vi "main.vi-simplified.vi"() -> ()   [LabVIEW 2023]
uses:
  state-machine-states.ctl
  sub-vi/csv-file-logging/filepath-selection.ctl
  tab-control-states.ctl
  <vilib>/DAQmx/read.llb/DAQmx Read (Analog DBL 1Chan 1Samp).vi
  <vilib>/DAQmx/create/channels.llb/DAQmx Create Channel (AI-Temperature-Thermocouple).vi
  <vilib>/DAQmx/miscellaneous.llb/DAQmx Fill In Error Info.vi
  bronkhorst_flow-bus/Bronkhorst FLOW-BUS/Public/Data/Measure/Read Measure (Direct).vi
  bronkhorst_flow-bus/Bronkhorst FLOW-BUS/Bronkhorst FLOW-BUS.lvlib
panel:
  in  "Datalogging options":T1={"Include Timestamp"=TRUE, "Include milliseconds"=FALSE, "data-precision"=3}
  in  "Stop":bool
  in  "pause":bool
  in  "exit":bool
  out "state":T2
  out "error out":errorcluster
  out "Status":string
  in  "Tab Control":enum32{"setup", "run", "graphs", "errors"}(tab)
  in  "Simulate Hardware":bool
  in  "Start":bool
  in  "MFC 1":refnum<visa-resource-name>="COM31"
  in  "MFC 2":refnum<visa-resource-name>="COM32"
  in  "MFM 3":refnum<visa-resource-name>="COM5"
  in  "MFM 4":refnum<visa-resource-name>="COM6"
  in  "TC1 Channel":tag="cDAQ1Mod1/ai0"
  in  "TC2 Channel":tag="cDAQ1Mod1/ai1"
  in  "Filepath Selection":T3={"Log Filepath Source"=enum."Application Relative (Auto)", "Log File Path (Manual)"=path "C:/Users/dheard/Documents/0002-labview-projects/ammonia-absorbsion-rig/data", "Log File Folder Name"="data", "log file name"="log", "Include Date in Filename"=TRUE, "Include Time in Filename"=TRUE}
  out "appended path for log file":path
  out "MFM4 (ml/min) 2":dbl caption="Measure Percentage"
  out "MFM3 (ml/min)":dbl caption="Measure Percentage"
  out "TC1 (degC)":dbl format="%0.2f"
  out "TC2 (degC)":dbl format="%0.2f"
  out "MFM Sensor History":dbl[][](graph)
  out "Temperature Sensor History":dbl[][](graph)
  out "errors":errorcluster
  in  "Clear Errors":bool
  # "Usage Instructions:\n\n1. Select \"setup\" tab, ensure correct \n    COM port & Channel for each device\n\n2. To start Data Aquisition press \"Start\" button\n\n3. View Graphs in \"graphs\" tab\n\n4. Pause and Unpause data aquisition with \"pause\" button\n\n5. To export data to Excel, right click on topmost graph view \n     and select:\n     - \"Export\" -> \"Export  Data to Excel\"\n     - Name & Save Excel file\n        (Note: All data will be exported not just \"active\" plots)\n\n\n6. To Clear sensor history press \"Stop\" button\n     - While stopped, setup controls are available\n\n7. To Exit program, click \"Exit\" Button\n\n8. If Error shows, attempt to remedy error then press\n     \"clear error\" button. Program will revert to Setup"
  # "Column Temp"
  # "Heater Temp"
  # "Percentage"
  # "Gas  \nOut"
  # "Nitrogen \nIn"
  # "Ammonia \nIn"
  # "Gas  \nOut"
  # "MFC2"
  # "MFM4"
  # "MFM3"
  # "MFC1"
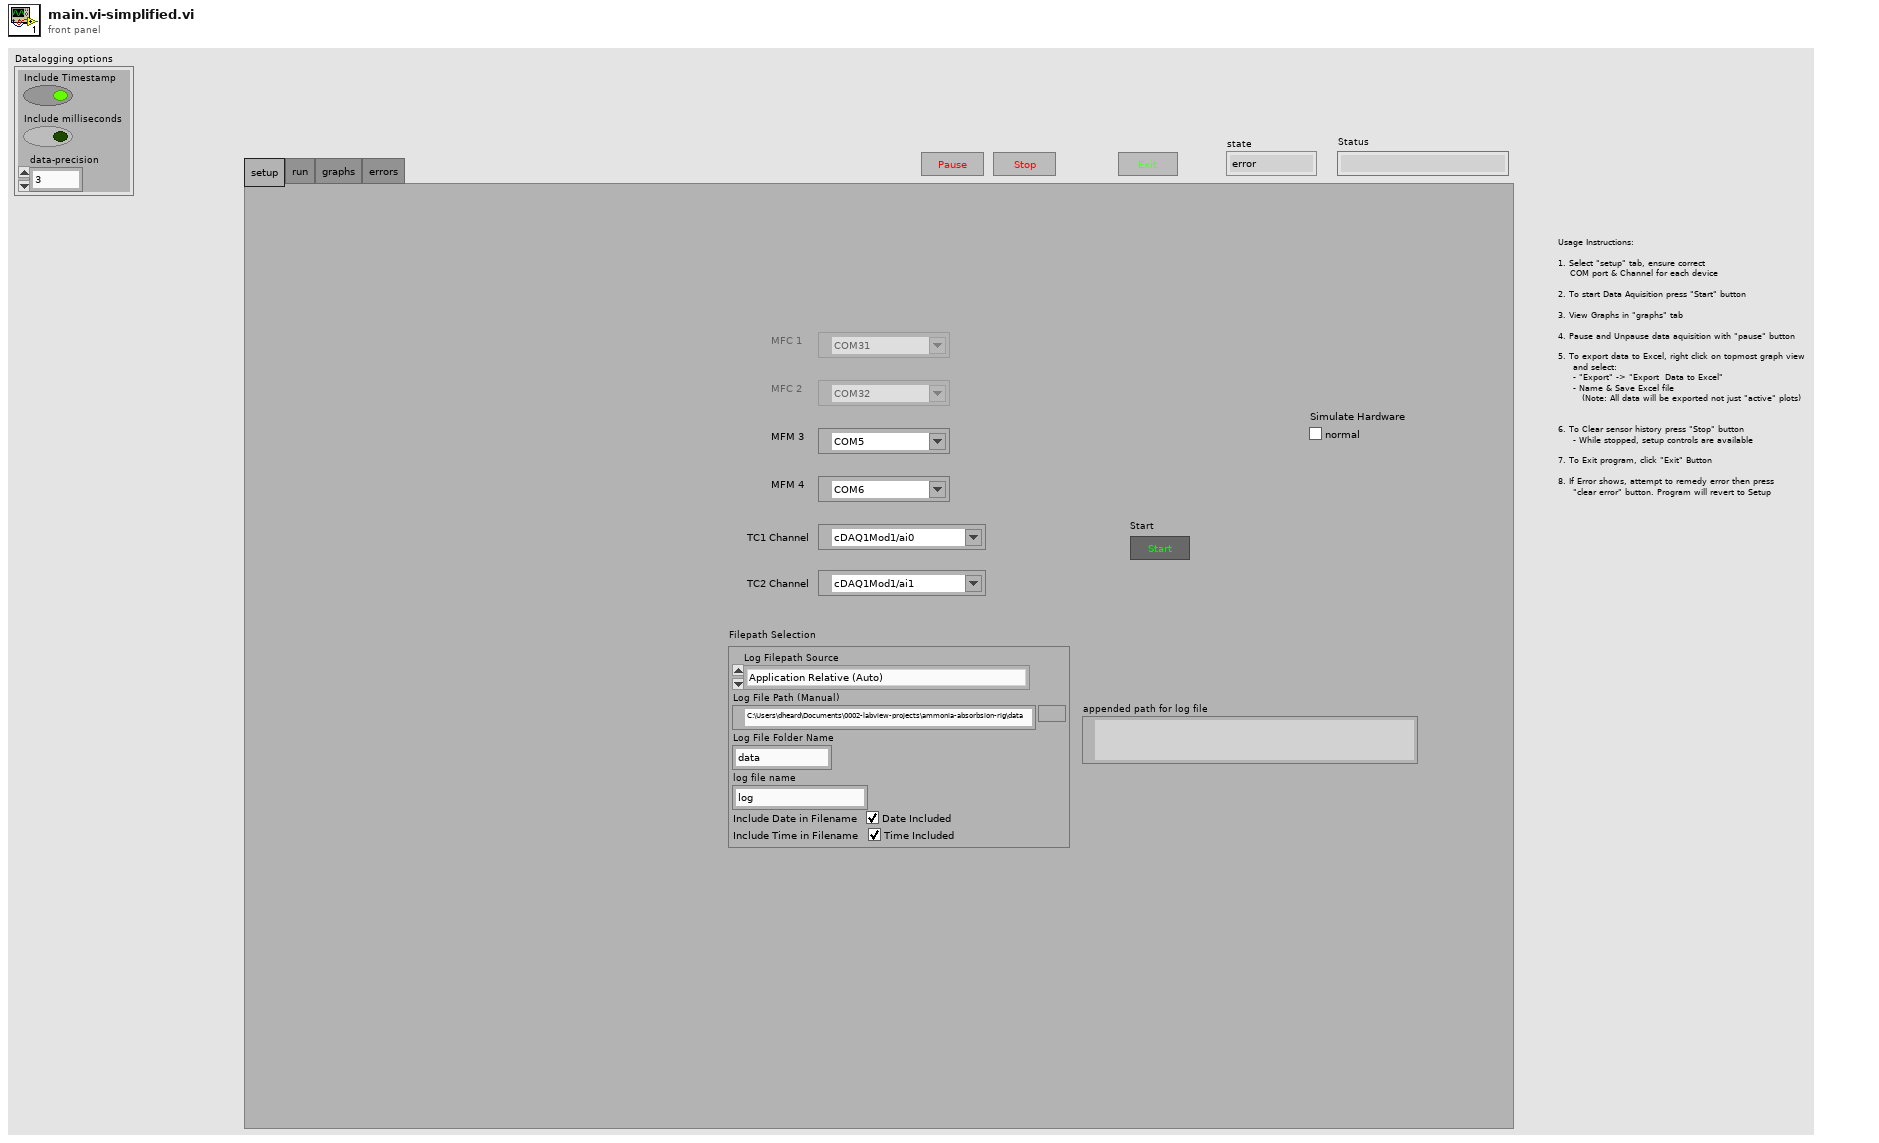
[diagram p1: front panel]
types:
  T1 = cluster{"Include Timestamp":bool, "Include milliseconds":bool, "data-precision":i32}
  T2 = typedef "state-machine-states.ctl" = enum16{"error", "wait", "init", "start", "run", "stop", "clear-error", "shutdown"}
  T3 = typedef "filepath-selection.ctl" = cluster{"Log Filepath Source":enum16{"Application Relative (Auto)", "VI Relative (Auto)", "Complete Path (Manual)"}, "Log File Path (Manual)":path, "Log File Folder Name":string, "log file name":string, "Include Date in Filename":bool, "Include Time in Filename":bool}
  T4 = enum8{"Enabled", "Disabled", "Disabled and Grayed Out"}
  T5 = typedef "tab-control-states.ctl" = enum32{"setup", "run", "graphs", "errors"}
  T6 = enum32{"BUS/RS232", "Analog input", "FLOW-BUS slave", "Valve close", "Controller idle", "Testing mode", "Tuning mode", "Setpoint 100%", "Valve fully open", "Calibration mode", "Analog slave", "Keyboard or FLOW-BUS setpoint", "Setpoint 0%", "FLOW-BUS analog slave", "(FPP) Range select mode", "(FPP) Manual start sensor select, automatic end sensor", "(FPP) Automatic start sensor select, manual end sensor", "(FPP) Automatic start and end sensor", "RS232 Setpoint", "RS232 broadcast mode", "Valve stearing (valve = setpoint)", "Analog valve stearing (valve = analog setpoint)", "Valve safe state"}
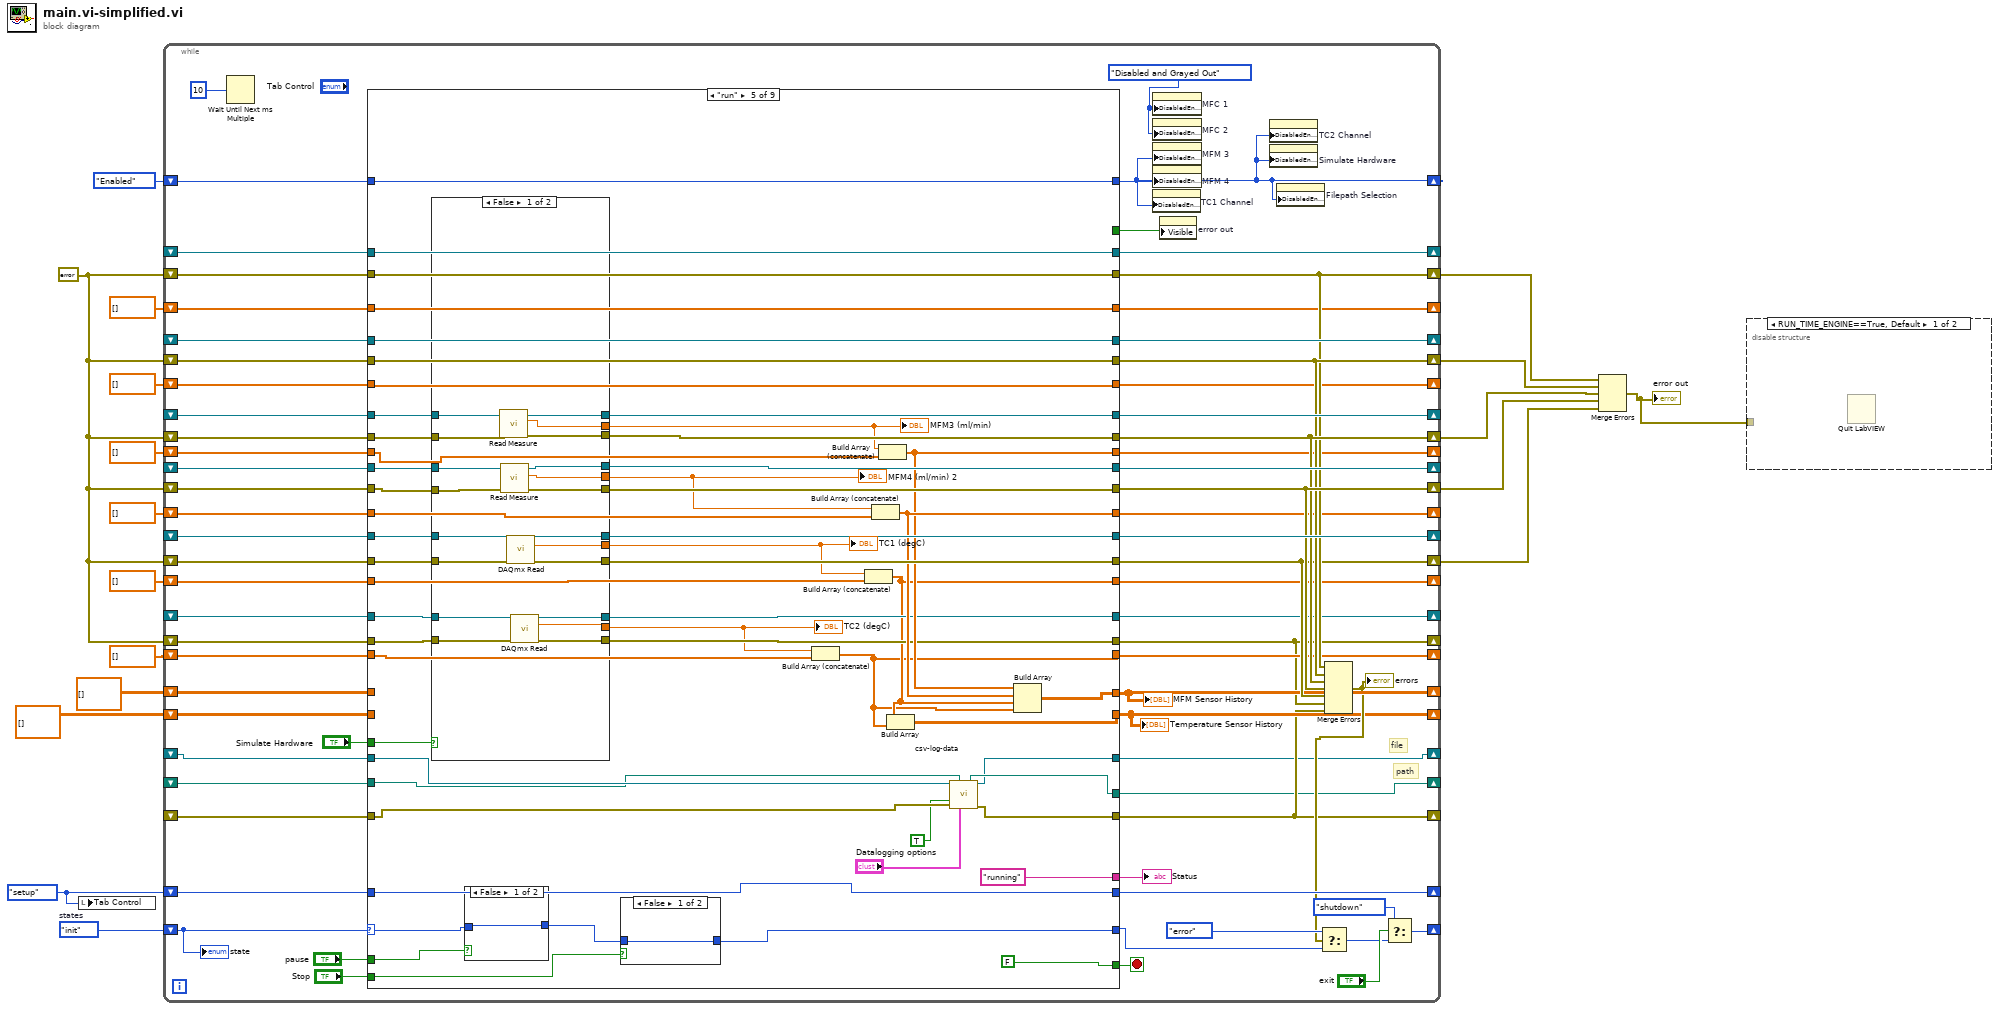
[diagram p0: block diagram]
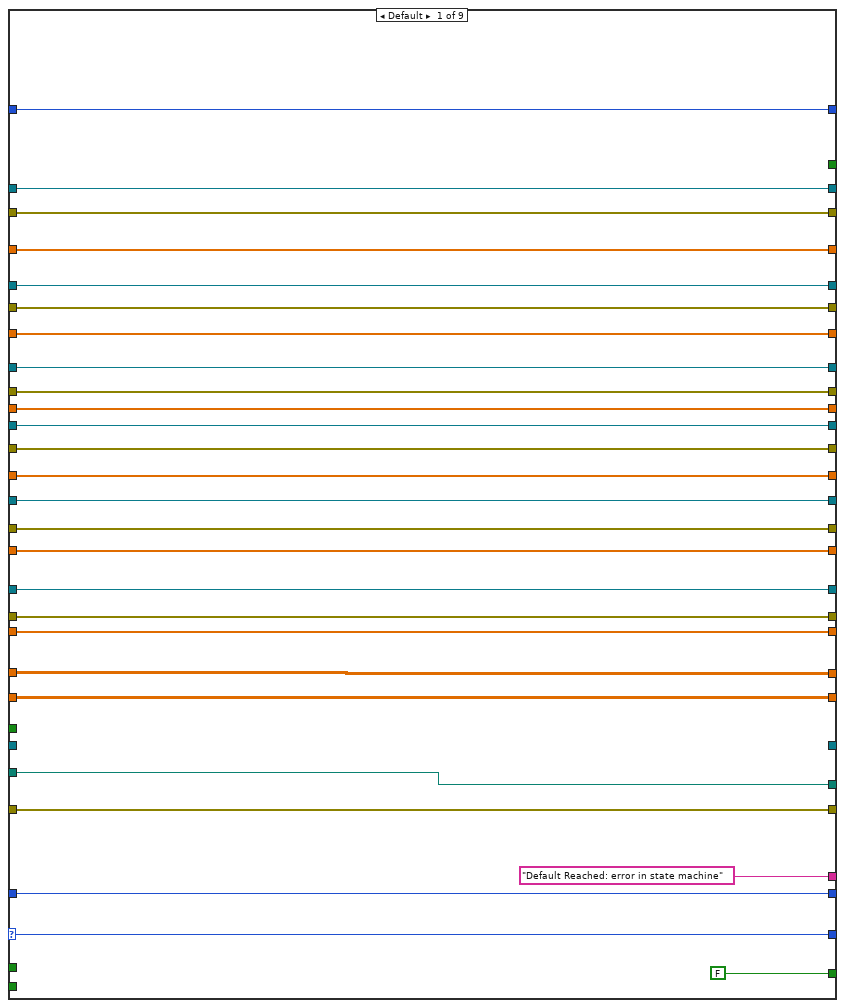
[diagram p3: hidden frame]
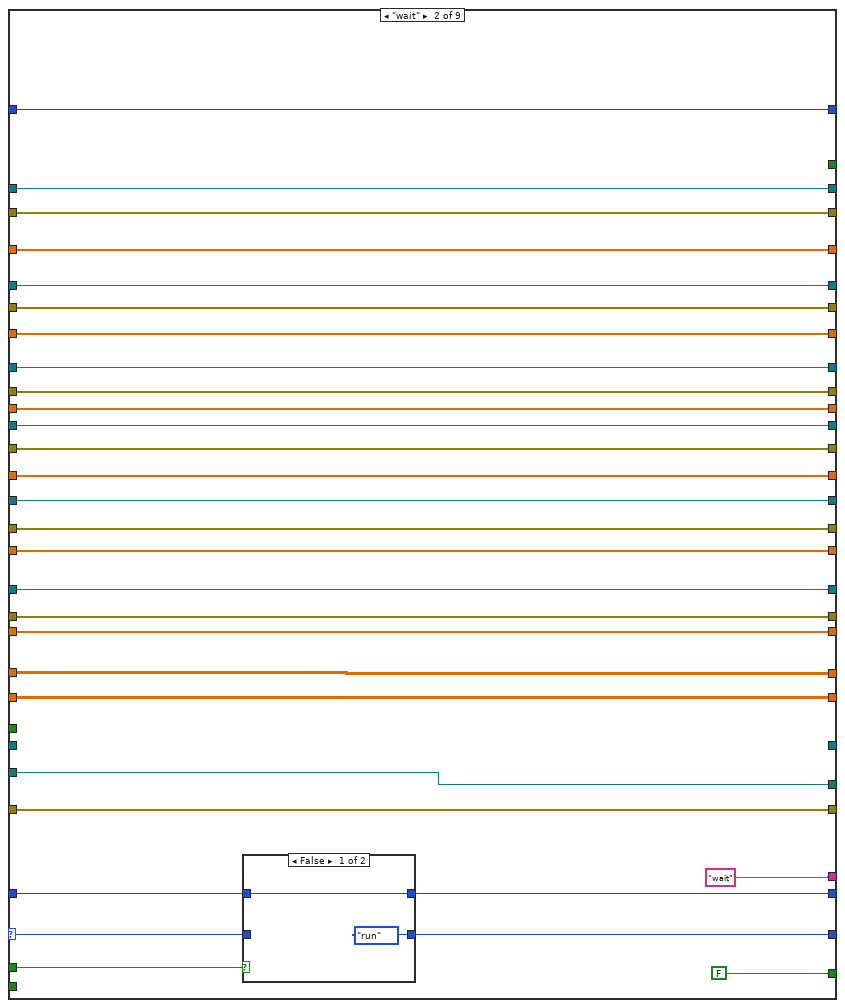
[diagram p4: hidden frame]
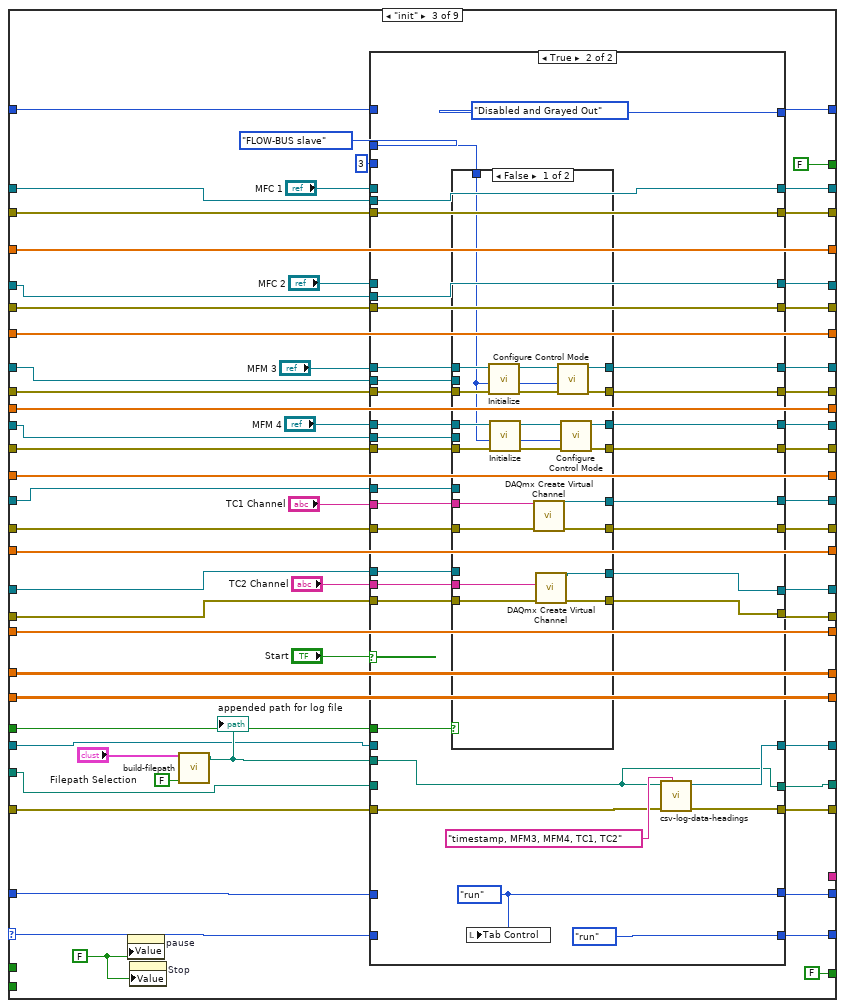
[diagram p6: hidden frame]
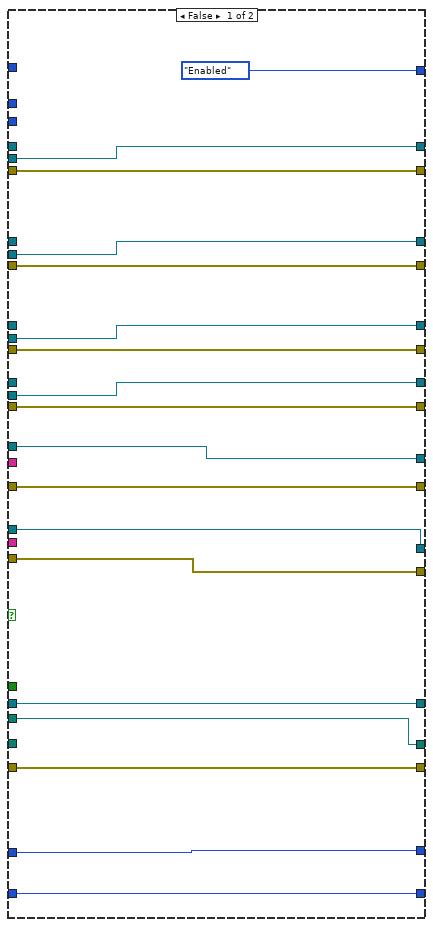
[diagram p7: hidden frame]
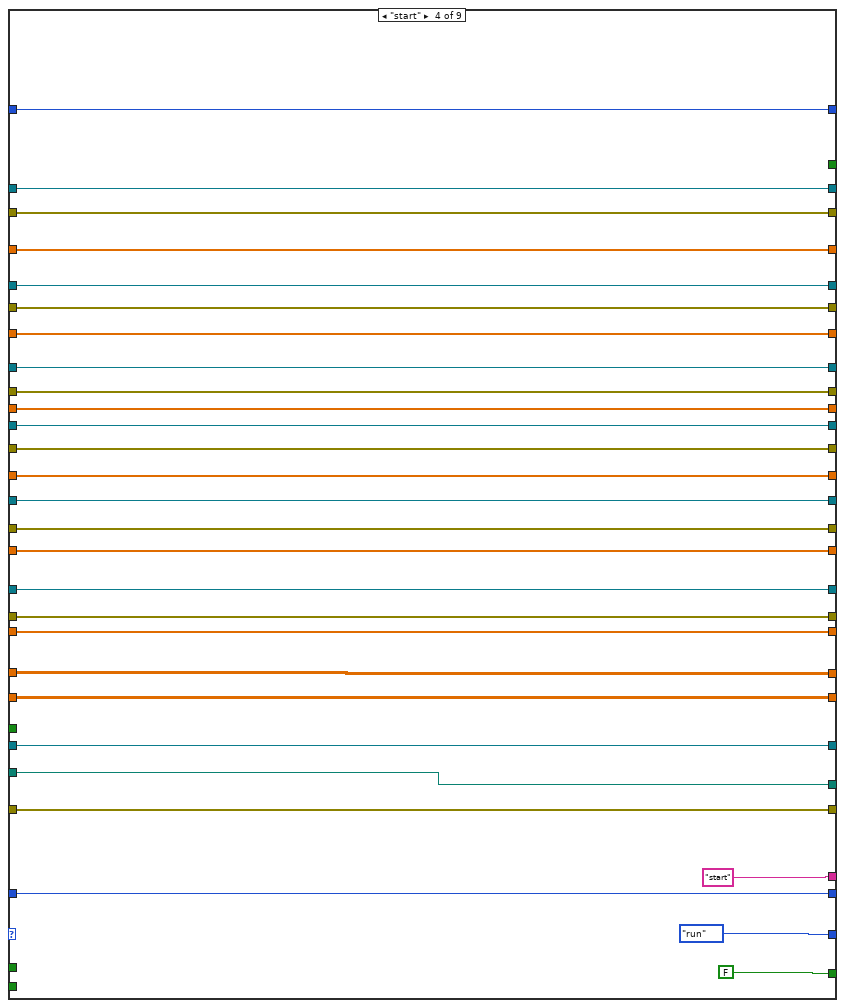
[diagram p9: hidden frame]
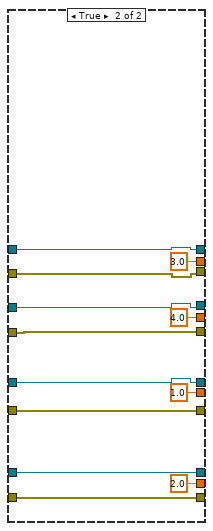
[diagram p10: hidden frame]
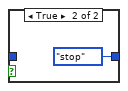
[diagram p11: hidden frame]
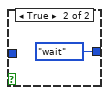
[diagram p12: hidden frame]
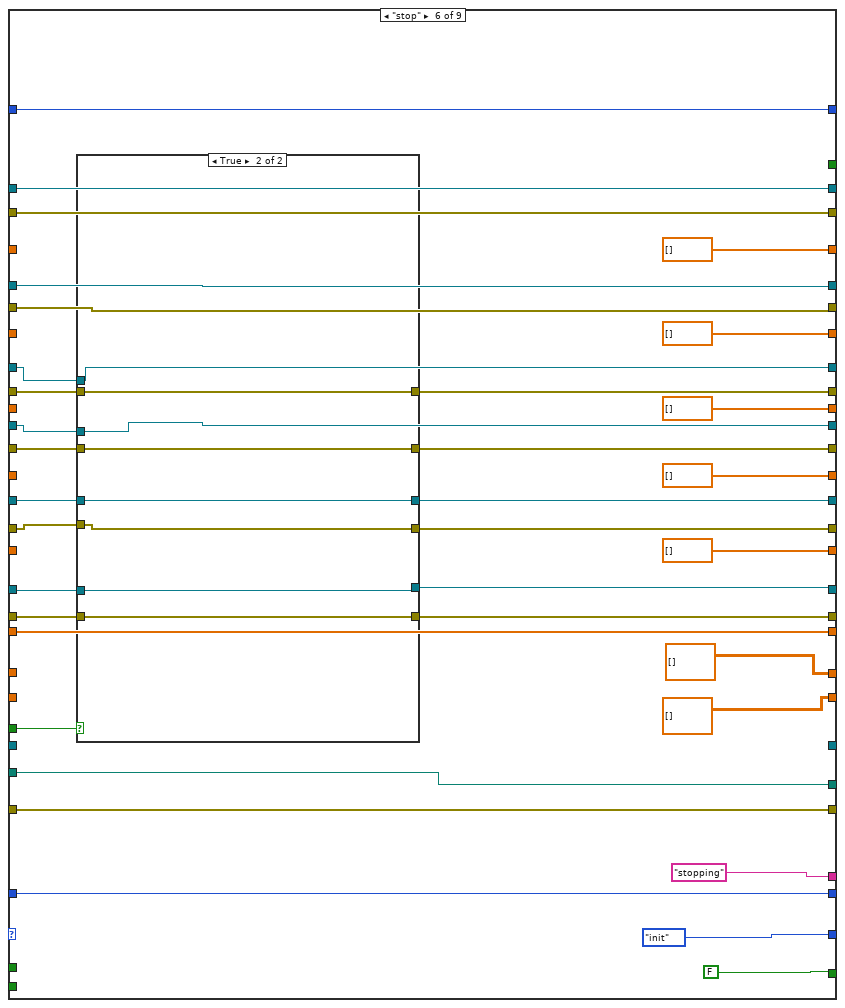
[diagram p13: hidden frame]
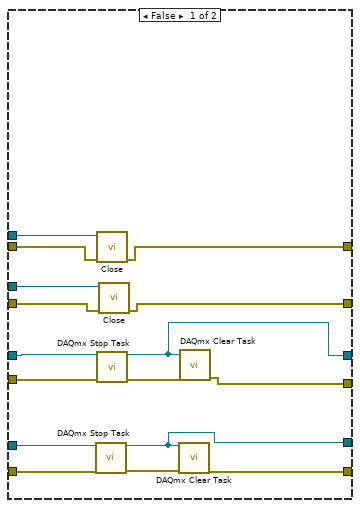
[diagram p14: hidden frame]
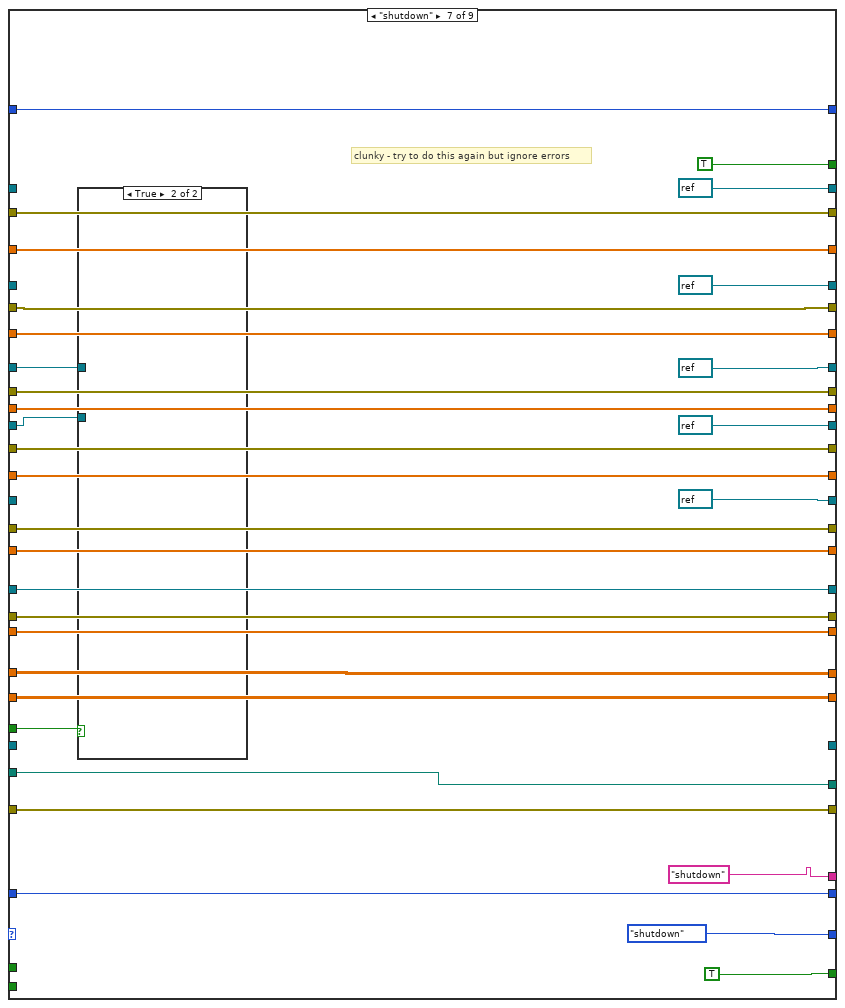
[diagram p15: hidden frame]
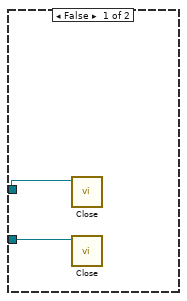
[diagram p16: hidden frame]
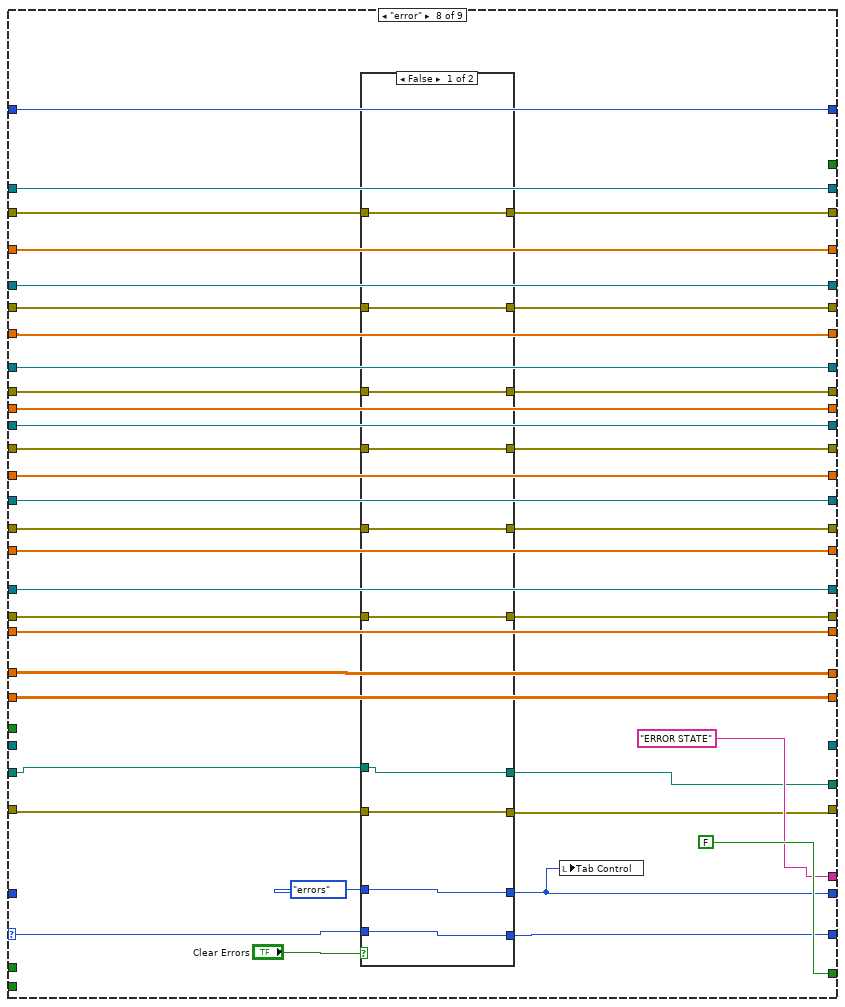
[diagram p17: hidden frame]
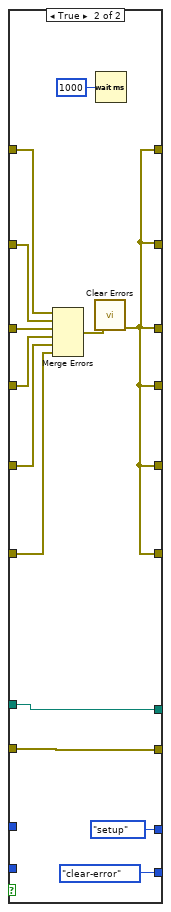
[diagram p18: hidden frame]
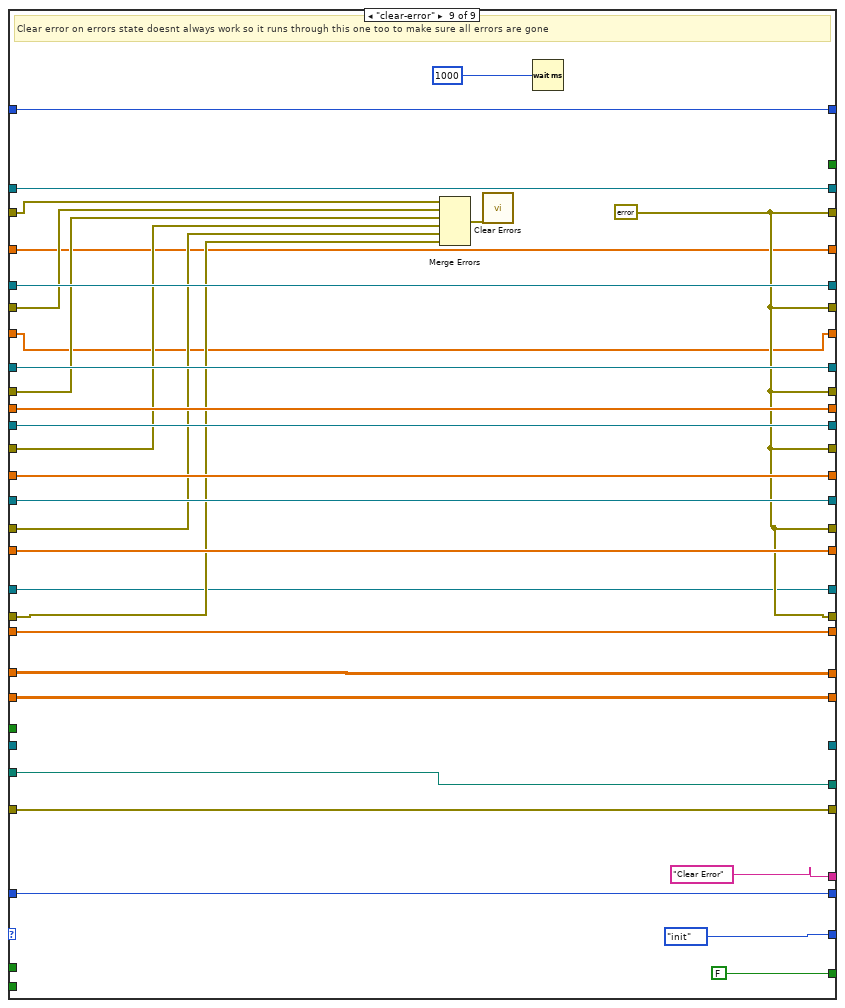
[diagram p19: hidden frame]
diagram:
  w3 = errorcluster {"status"=FALSE, "code"=0, "source"=""} ("error out")
  w13 = state-machine-states."init"  # states
  w11 = tab-control-states."setup" ("Tab Control")
  n1 = local write "Tab Control"(w11) -> ()
  n2 = while {
    shift-right: [w68] -> _
    shift-left: w11 -> [w58]
    shift-right: [w84] -> _
    shift-left: _ -> [w76]
    shift-right: [w61] -> w18
    shift-left: w3 -> [w80]
    shift-right: [w83] -> _
    shift-left: _ -> [w75]
    shift-right: [w62] -> w17
    shift-left: w3 -> [w79]
    shift-right: [w82] -> _
    shift-left: _ -> [w74]
    shift-right: [w63] -> w16
    shift-left: w3 -> [w78]
    shift-right: [w81] -> _
    shift-left: _ -> [w73]
    shift-right: [w64] -> w15
    shift-left: w3 -> [w77]
    shift-right: [w72] -> _
    shift-left: _ -> [w71]
    shift-right: [w60] -> w14
    shift-left: w3 -> [w70]
    shift-right: [w55] -> _
    shift-left: w13 -> [w66]
    shift-right: [w22] -> _
    shift-left: T4."Enabled" ("Disabled") -> [w59]
    shift-right: [w49] -> _
    shift-left: sgl[] [] -> [w48]
    shift-right: [w47] -> _
    shift-left: dbl[] [] -> [w46]
    shift-right: [w45] -> _
    shift-left: sgl[] [] -> [w44]
    shift-right: [w36] -> _
    shift-left: dbl[] [] -> [w43]
    shift-right: [w37] -> _
    shift-left: dbl[] [] -> [w42]
    shift-right: [w41] -> _
    shift-left: dbl[][] [] -> [w40]
    shift-right: [w35] -> _
    shift-left: _ -> [w34]
    shift-right: [w29] -> _
    shift-left: w3 -> [w33]
    shift-right: [w30] -> _
    shift-left: dbl[] [] -> [w32]
    shift-right: [w28] -> _
    shift-left: dbl[][] [] -> [w27]
    shift-right: [w24] -> _
    shift-left: _ -> [w25]
    shift-right: [w19] -> _
    shift-left: _ -> [w23]
    shift-right: [w20] -> _
    shift-left: _ -> [w21]
    stop <- w53 stop-if-true
    w38 = T4."Disabled and Grayed Out" ("Disabled")
    # "file"
    # "path"
    n3 = Wait Until Next ms Multiple(millisecond multiple=u32 10) -> ()  [unwired: 1 out]
    n4 = case shown="\"run\"" w66 {
      selector: w66 -> [w99 w125 w204 _ w356 _ _ w517 _]
      tunnel: [w101 w126 w173 w304 w353 w437 w490 w515 w564] -> w68
      tunnel: w58 -> [w101 w127 w205 w304 w353 w437 w490 _ w564]
      tunnel: [w111 w141 w185 w314 w338 w425 refnum<visa-resource-name> refnum ("VISA resource name out") w531 w584] -> w84
      tunnel: [w110 w140 w186 w313 w339 w417 w485 w509 w562] -> w61
      tunnel: [w108 w131 w191 w312 w336 w426 refnum<visa-resource-name> refnum ("VISA resource name out") w530 w583] -> w83
      tunnel: [w109 w132 w192 w311 w340 w416 w479 w508 w562] -> w62
      tunnel: [w107 w133 w197 w310 w361 w430 refnum<visa-resource-name> refnum ("VISA resource name out") w529 w582] -> w82
      tunnel: [w106 w134 w198 w309 w362 w431 w478 w507 w562] -> w63
      tunnel: [w105 w135 w201 w308 w358 w428 refnum<visa-resource-name> refnum ("VISA resource name out") w528 w581] -> w81
      tunnel: [w104 w136 w202 w307 w357 w427 w477 w506 w562] -> w64
      tunnel: w80 -> [w110 w140 w188 w313 w339 w417 w485 w514 w570]
      tunnel: w79 -> [w109 w132 w194 w311 w340 w416 w479 w513 w569]
      tunnel: w78 -> [w106 w134 w196 w309 w363 w432 w478 w512 w568]
      tunnel: w77 -> [w104 w136 w200 w307 w359 w429 w477 w511 w567]
      tunnel: w76 -> [w111 w141 w177 w314 w338 w425 _ w531 w584]
      tunnel: w75 -> [w108 w131 w178 w312 w336 w426 _ w530 w583]
      tunnel: w74 -> [w107 w133 w176 w310 w364 w430 w487 w529 w582]
      tunnel: w73 -> [w105 w135 w179 w308 w360 w428 w486 w528 w581]
      tunnel: [w103 w137 w181 w306 w366 w433 refnum<k21> refnum ("task out") w527 w580] -> w72
      tunnel: w71 -> [w103 w137 w184 w306 w368 w436 _ w527 w580]
      tunnel: [w102 w138 w180 w305 w365 w434 w476 w505 w562] -> w60
      tunnel: w70 -> [w102 w138 w182 w305 w367 w435 w476 w510 w566]
      tunnel: ["Default Reached: error in state machine" ("Status") "wait" ("Status") _ "start" ("Status") "running" ("Status") "stopping" ("Status") "shutdown" ("Status") "ERROR STATE" ("Status") "Clear Error" ("Status")] -> w67
      tunnel: [w99 w124 w156 state-machine-states."run" ("Enum") w349 state-machine-states."init" ("Enum") state-machine-states."shutdown" ("Enum") w518 state-machine-states."init"] -> w51
      tunnel: [FALSE ("x") FALSE ("x") FALSE ("x") FALSE ("x") FALSE ("x") FALSE ("x") TRUE ("x") FALSE ("x") FALSE ("x")] -> w53
      tunnel: [w97 w129 w175 w300 w354 w422 w488 w525 w578] -> w22
      tunnel: w59 -> [w97 w129 w174 w300 w354 w422 w488 w525 w578]
      tunnel: "pause" -> [_ w128 _ _ w352 _ _ _ _]
      tunnel: "Stop" -> [_ _ _ _ w351 _ _ _ _]
      tunnel: [w94 w121 w169 w299 w323 dbl[][] [] w474 w522 w575] -> w41
      tunnel: [w96 w123 w171 w298 w344 sgl[] [] w472 w523 w576] -> w49
      tunnel: w48 -> [w96 w123 w171 w298 w346 _ w472 w523 w576]
      tunnel: [w93 w120 w168 w296 w328 dbl[] [] w473 w521 w574] -> w47
      tunnel: w46 -> [w93 w120 w168 w296 w345 _ w473 w521 w574]
      tunnel: [w87 w116 w158 w290 w327 dbl[][] [] w466 w498 w559] -> w28
      tunnel: [w95 w122 w170 w297 w341 sgl[] [] w471 w524 w577] -> w45
      tunnel: w44 -> [w95 w122 w170 w297 w342 _ w471 w524 w577]
      tunnel: [w91 w114 w160 w291 w337 dbl[] [] w464 w500 w557] -> w36
      tunnel: w43 -> [w91 w114 w160 w291 w337 _ w464 w500 w557]
      tunnel: w42 -> [w92 w115 w161 w292 w335 _ w465 w501 w558]
      tunnel: w40 -> [w94 w121 w169 w299 _ _ w474 w522 w575]
      tunnel: [_ _ FALSE ("Visible") _ _ _ TRUE ("Visible") _ _] -> w39
      tunnel: [w92 w115 w161 w292 w335 dbl[] [] w465 w501 w558] -> w37
      tunnel: [w90 w119 w165 w295 w331 w410 w469 w504 w561] -> w35
      tunnel: w34 -> [w90 w119 w164 w295 w332 w413 w469 w504 w561]
      tunnel: [w89 w118 w163 w294 w333 w411 w468 w502 w562] -> w29
      tunnel: w33 -> [w89 w118 w162 w294 w334 w412 w468 w503 w563]
      tunnel: w32 -> [w88 w117 w159 w293 w329 w409 w467 w499 w560]
      tunnel: [w88 w117 w159 w293 w324 w409 w467 w499 w560] -> w30
      tunnel: w27 -> [w87 w116 w158 w290 _ _ w466 w498 w559]
      tunnel: "Simulate Hardware" -> [_ _ w155 _ w326 w407 w463 _ _]
      tunnel: [w85 w112 w154 w289 w317 w405 w461 w495 w555] -> w24
      tunnel: w25 -> [w85 w112 w153 w289 w318 w405 w461 w494 w555]
      tunnel: [w86 w113 w152 w288 w320 w406 w462 w497 w556] -> w19
      tunnel: w23 -> [w86 w113 w146 w288 w321 w406 w462 w496 w556]
      tunnel: w21 -> [_ _ w148 w287 w322 _ _ _ _]
      tunnel: [_ _ w147 w287 w319 _ _ _ _] -> w20
      frame Default {
      }
      frame "wait" {
        n5 = case shown="False" w128 {
          tunnel: w125 -> [_ w144]
          tunnel: w127 -> [w143 w145]
          tunnel: [w143 w145] -> w126
          tunnel: [state-machine-states."run" w144] -> w124
          frame False {
          }
          frame True {
          }
        }
      }
      frame "init" {
        w172 = FALSE ("pause")
        n6 = property on="pause" class="Bool (strict)"("Value"=w172) -> ()  [unwired: 2 in, 2 out]
        n7 = property on="Stop" class="Bool (strict)"("Value"=w172) -> ()  [unwired: 2 in, 2 out]
        n8 = call "build-filepath.vi"("Include Seconds in Filename"=FALSE, "Filepath Selection"="Filepath Selection") -> ("appended path for log file"=w151:path)  [unwired: 8 in, 1 out]
        "appended path for log file" <- w151
        n9 = case shown="True" "Start" {
          tunnel: [w214 w242] -> w173
          tunnel: w205 -> [w214 _]
          tunnel: w204 -> [w213 _]
          tunnel: [w213 state-machine-states."run" ("Enum")] -> w156
          tunnel: [w218 w257] -> w202
          tunnel: [w223 w256] -> w201
          tunnel: w200 -> [w218 w255]
          tunnel: "MFM 4" -> [_ w254]
          tunnel: [w217 w253] -> w198
          tunnel: [w220 w252] -> w197
          tunnel: w196 -> [w217 w251]
          tunnel: "MFM 3" -> [_ w250]
          tunnel: w194 -> [w216 w240]
          tunnel: "MFC 2" -> [_ _]
          tunnel: [w216 w240] -> w192
          tunnel: [w222 w241] -> w191
          tunnel: T6."FLOW-BUS slave" ("Control Mode (0: BUS/RS232)") -> [_ w246]
          tunnel: u8 3 ("Node (3)") -> [_ _]
          tunnel: w188 -> [w215 w239]
          tunnel: "MFC 1" -> [_ _]
          tunnel: [w215 w239] -> w186
          tunnel: [w221 w238] -> w185
          tunnel: w184 -> [w211 w230]
          tunnel: "TC1 Channel" -> [_ w244]
          tunnel: w182 -> [w219 w249]
          tunnel: [w211 w248] -> w181
          tunnel: [w219 w247] -> w180
          tunnel: w179 -> [w223 w231]
          tunnel: w178 -> [w222 w241]
          tunnel: w177 -> [w221 w238]
          tunnel: w176 -> [w220 w232]
          tunnel: [T4."Enabled" ("Disabled") T4."Disabled and Grayed Out" ("Disabled")] -> w175
          tunnel: w174 -> [_ _]
          tunnel: "TC2 Channel" -> [_ w237]
          tunnel: [w210 w236] -> w165
          tunnel: w164 -> [w210 w229]
          tunnel: [w209 w235] -> w163
          tunnel: w162 -> [w209 w234]
          tunnel: w155 -> [_ w233]
          tunnel: w151 -> [w207 w224]
          tunnel: [w208 w226] -> w154
          tunnel: w153 -> [w208 w227]
          tunnel: [w207 w224] -> w152
          tunnel: w148 -> [w206 _]
          tunnel: [w206 w225] -> w147
          tunnel: w146 -> [_ _]
          frame False {
          }
          frame True {
            w242 = tab-control-states."run" ("Tab Control")
            n10 = case shown="False" w233 {
              tunnel: [w278 w280] -> w257
              tunnel: [w277 w285] -> w256
              tunnel: w255 -> [w276 w280]
              tunnel: w254 -> [w275 _]
              tunnel: [w272 w284] -> w253
              tunnel: [w271 w286] -> w252
              tunnel: w251 -> [w270 w284]
              tunnel: w250 -> [w269 _]
              tunnel: w249 -> [w266 w281]
              tunnel: [w265 w283] -> w248
              tunnel: [w264 w281] -> w247
              tunnel: w246 -> [w263 _]
              tunnel: w244 -> [w262 _]
              tunnel: w237 -> [w261 _]
              tunnel: [w260 w282] -> w236
              tunnel: [w259 w279] -> w235
              tunnel: w234 -> [w258 w279]
              tunnel: w232 -> [_ w286]
              tunnel: w231 -> [_ w285]
              tunnel: w230 -> [_ w283]
              tunnel: w229 -> [_ w282]
              frame False {
                n11 = call "Initialize.vi"("error in (no error)"=w270, "VISA resource name"=w269) -> ("error out"=w268:errorcluster, "VISA resource name out"=w267:refnum<visa-resource-name>)  [unwired: 8 in]
                n12 = call "Initialize.vi"("error in (no error)"=w276, "VISA resource name"=w275) -> ("error out"=w274:errorcluster, "VISA resource name out"=w273:refnum<visa-resource-name>)  [unwired: 8 in]
                n13 = call-poly <vilib>:"DAQmx Create Virtual Channel.vi"("physical channels"=w262, "error in"=w266) -> ("task out"=w265:refnum<k21>, "error out"=w264:errorcluster)  [unwired: 12 in]
                n14 = call-poly <vilib>:"DAQmx Create Virtual Channel.vi"("physical channels"=w261, "error in"=w258) -> ("task out"=w260:refnum<k21>, "error out"=w259:errorcluster)  [unwired: 12 in]
                n15 = call "Configure Control Mode.vi"("error in (no error)"=w268, "Control Mode (0: BUS/RS232)"=w263, "VISA resource name"=w267) -> ("error out"=w272:errorcluster, "VISA resource name out"=w271:refnum<visa-resource-name>)  [unwired: 7 in]
                n16 = call "Configure Control Mode.vi"("error in (no error)"=w274, "Control Mode (0: BUS/RS232)"=w263, "VISA resource name"=w273) -> ("error out"=w278:errorcluster, "VISA resource name out"=w277:refnum<visa-resource-name>)  [unwired: 7 in]
              }
              frame True {
              }
            }
            n17 = local write "Tab Control"(w242) -> ()
            n18 = call "csv-log-data-headings.vi"("CSV Data Headings"="timestamp, MFM3, MFM4, TC1, TC2", "error in (no error)"=w227, "Log File Path"=w224) -> ("error out"=w226:errorcluster, "Byte Stream File out"=w225:refnum<file>)  [unwired: 6 in, 1 out]
          }
        }
      }
      frame "start" {
      }
      frame "run" {
        n19 = case shown="False" w326 {
          tunnel: w368 -> [w388 w395]
          tunnel: w367 -> [w387 w396]
          tunnel: [w386 w395] -> w366
          tunnel: [w385 w396] -> w365
          tunnel: w364 -> [w384 w391]
          tunnel: w363 -> [w383 w390]
          tunnel: [w382 w390] -> w362
          tunnel: [w381 w391] -> w361
          tunnel: w360 -> [w380 w389]
          tunnel: w359 -> [w379 w394]
          tunnel: [w378 w389] -> w358
          tunnel: [w377 w394] -> w357
          tunnel: [w376 sgl 4.0 ("Measure Direct")] -> w348
          tunnel: [w375 1.0 ("data")] -> w347
          tunnel: [w374 sgl 3.0 ("Measure Direct")] -> w343
          tunnel: w334 -> [w373 w399]
          tunnel: [w372 w399] -> w333
          tunnel: w332 -> [w371 w400]
          tunnel: [w370 w400] -> w331
          tunnel: [w369 2.0 ("data")] -> w330
          frame False {
            n20 = call-poly "Read Measure.vi"("error in (no error)"=w383, "VISA resource name"=w384) -> ("error out"=w382:errorcluster, "Measure Direct"=w374:sgl, "VISA resource name out"=w381:refnum<visa-resource-name>)  [unwired: 7 in]
            n21 = call-poly "Read Measure.vi"("error in (no error)"=w379, "VISA resource name"=w380) -> ("error out"=w377:errorcluster, "Measure Direct"=w376:sgl, "VISA resource name out"=w378:refnum<visa-resource-name>)  [unwired: 7 in]
            n22 = call-poly <vilib>:"DAQmx Read.vi"("task/channels in"=w388, "error in"=w387) -> ("task out"=w386:refnum<k21>, "data"=w375:dbl, "error out"=w385:errorcluster)  [unwired: 11 in]
            n23 = call-poly <vilib>:"DAQmx Read.vi"("task/channels in"=w371, "error in"=w373) -> ("task out"=w370:refnum<k21>, "data"=w369:dbl, "error out"=w372:errorcluster)  [unwired: 11 in]
          }
          frame True {
          }
        }
        "TC1 (degC)" <- w347
        "MFM3 (ml/min)" <- w343
        "MFM4 (ml/min) 2" <- w348
        "TC2 (degC)" <- w330
        n24 = case shown="False" w352 {
          tunnel: w356 -> [w403 _]
          tunnel: [w403 state-machine-states."wait"] -> w350
          frame False {
          }
          frame True {
          }
        }
        n25 = case shown="False" w351 {
          tunnel: w350 -> [w401 _]
          tunnel: [w401 state-machine-states."stop"] -> w349
          frame False {
          }
          frame True {
          }
        }
        n26 = Build Array (concatenate)(w330, w329) -> (w324:dbl[])
        n27 = Build Array (concatenate)(w347, w345) -> (w328:dbl[])
        n28 = Build Array (concatenate)(w348, w346) -> (w344:sgl[])
        n29 = Build Array (concatenate)(w343, w342) -> (w341:sgl[])
        n30 = Build Array(w328, w324) -> (w327:dbl[][])
        n31 = call "csv-log-data.vi"("log file Byte Stream File in"=w322, "log file path"=w321, "File Open?"=TRUE ("append to file? (new file:F)"), "error in (no error)"=w318, "Datalogging options"="Datalogging options") -> ("log file path"=w320:path, "log file Byte Stream File out"=w319:refnum<file>, "error out"=w317:errorcluster)  [unwired: 6 in, 2 out]
        n32 = Build Array(w341, w344, w328, w324) -> (w323:dbl[][])
      }
      frame "stop" {
        n33 = case shown="True" w407 {
          tunnel: w436 -> [w453 w457]
          tunnel: w435 -> [w452 w458]
          tunnel: [w451 w458] -> w434
          tunnel: [w450 w457] -> w433
          tunnel: w432 -> [w449 w455]
          tunnel: [w448 w455] -> w431
          tunnel: w430 -> [w447 _]
          tunnel: w429 -> [w446 w456]
          tunnel: w428 -> [w445 _]
          tunnel: [w444 w456] -> w427
          tunnel: w413 -> [w442 w459]
          tunnel: w412 -> [w441 w460]
          tunnel: [w440 w460] -> w411
          tunnel: [w439 w459] -> w410
          frame False {
            n34 = call <vilib>:"DAQmx Stop Task.vi"("task/channels in"=w442, "error in"=w441) -> ("task out"=w439:refnum<k21>, "error out"=w443:errorcluster)  [unwired: 12 in]
            n35 = call "Close.vi"("error in (no error)"=w449, "VISA resource name"=w447) -> ("error out"=w448:errorcluster)  [unwired: 9 in]
            n36 = call <vilib>:"DAQmx Stop Task.vi"("task/channels in"=w453, "error in"=w452) -> ("task out"=w450:refnum<k21>, "error out"=w454:errorcluster)  [unwired: 12 in]
            n37 = call "Close.vi"("error in (no error)"=w446, "VISA resource name"=w445) -> ("error out"=w444:errorcluster)  [unwired: 9 in]
            n38 = call <vilib>:"DAQmx Clear Task.vi"("task in"=w439, "error in"=w443) -> ("error out"=w440:errorcluster)  [unwired: 13 in]
            n39 = call <vilib>:"DAQmx Clear Task.vi"("task in"=w450, "error in"=w454) -> ("error out"=w451:errorcluster)  [unwired: 13 in]
          }
          frame True {
          }
        }
      }
      frame "shutdown" {
        # "clunky - try to do this again but ignore errors"
        n40 = case shown="True" w463 {
          tunnel: w487 -> [w493 _]
          tunnel: w486 -> [w492 _]
          frame False {
            n41 = call "Close.vi"("VISA resource name"=w493) -> ()  [unwired: 10 in, 1 out]
            n42 = call "Close.vi"("VISA resource name"=w492) -> ()  [unwired: 10 in, 1 out]
          }
          frame True {
          }
        }
      }
      frame "error" {
        n43 = case shown="False" "Clear Errors" {
          tunnel: [w540 state-machine-states."clear-error"] -> w518
          tunnel: w517 -> [w540 _]
          tunnel: tab-control-states."errors" ("Tab Control") -> [w541 _]
          tunnel: [w541 tab-control-states."setup" ("Tab Control")] -> w515
          tunnel: w514 -> [w539 w552]
          tunnel: w513 -> [w538 w551]
          tunnel: w512 -> [w537 w550]
          tunnel: w511 -> [w536 w549]
          tunnel: w510 -> [w535 w548]
          tunnel: [w539 w544] -> w509
          tunnel: [w538 w544] -> w508
          tunnel: [w537 w544] -> w507
          tunnel: [w536 w544] -> w506
          tunnel: [w535 w544] -> w505
          tunnel: w503 -> [w534 w545]
          tunnel: [w534 w544] -> w502
          tunnel: [w533 w543] -> w497
          tunnel: w496 -> [w533 w543]
          tunnel: [w532 w542] -> w495
          tunnel: w494 -> [w532 w542]
          frame False {
          }
          frame True {
            n44 = Merge Errors(w552, w551, w550, w549, w548, w545) -> (w547:errorcluster)
            n45 = call <vilib>:"Clear Errors.vi"("error in (no error)"=w547) -> ("error out"=w544:errorcluster)  [unwired: 5 in, 1 out]
            n46 = Wait (ms)(milliseconds to wait=u32 1000) -> ()  [unwired: 1 out]
          }
        }
        n47 = local write "Tab Control"(w515) -> ()
      }
      frame "clear-error" {
        w562 = errorcluster {"status"=FALSE, "code"=0, "source"=""} ("error out")
        # "Clear error on errors state doesnt always work so it runs through this one too to make sure all errors are gone"
        n48 = Merge Errors(w570, w569, w568, w567, w566, w563) -> (w572:errorcluster)
        n49 = call <vilib>:"Clear Errors.vi"("error in (no error)"=w572) -> ()  [unwired: 5 in, 2 out]
        n50 = Wait (ms)(milliseconds to wait=u32 1000) -> ()  [unwired: 1 out]
      }
    }
    "Status" <- w67
    "MFM Sensor History" <- w41
    "Temperature Sensor History" <- w28
    n51 = property on="TC1 Channel" class="DAQmxName"("DisabledEnum"=w22) -> ()  [unwired: 2 in, 2 out]
    n52 = property on="MFC 1" class="VISAName"("DisabledEnum"=w38) -> ()  [unwired: 2 in, 2 out]
    n53 = property on="MFC 2" class="VISAName"("DisabledEnum"=w38) -> ()  [unwired: 2 in, 2 out]
    n54 = property on="MFM 3" class="VISAName"("DisabledEnum"=w22) -> ()  [unwired: 2 in, 2 out]
    n55 = property on="MFM 4" class="VISAName"("DisabledEnum"=w22) -> ()  [unwired: 2 in, 2 out]
    n56 = property on="error out" class="Clust (strict)"("Visible"=w39) -> ()  [unwired: 2 in, 2 out]
    n57 = property on="TC2 Channel" class="DAQmxName"("DisabledEnum"=w22) -> ()  [unwired: 2 in, 2 out]
    n58 = property on="Simulate Hardware" class="Bool (strict)"("DisabledEnum"=w22) -> ()  [unwired: 2 in, 2 out]
    n59 = property on="Filepath Selection" class="Clust (strict)"("DisabledEnum"=w22) -> ()  [unwired: 2 in, 2 out]
    n60 = Merge Errors(w61, w62, w63, w64, w60, w29, w24) -> (w31:errorcluster)
    "errors" <- w31
    n61 = Select(t=state-machine-states."error", s=w31, f=w51) -> (s? t:f=w50:T2)
    n62 = Select(t=state-machine-states."shutdown", s="exit", f=w50) -> (s? t:f=w55:T2)
    "state" <- w66
  }
  n63 = Merge Errors(w18, w17, w16, w15, w14) -> (w1:errorcluster)
  "error out" <- w1
  n64 = disable-structure shown="RUN_TIME_ENGINE==True, Default" {
    disable-tunnel: w1 -> [_ _]
    frame condition #0 {
      n65 = Quit LabVIEW() -> ()  [unwired: 1 in]
    }
    frame condition #1 (active) {
    }
  }
